vi "一个反馈计算误差.vi"(6 "第几组":i32, 7 "选择?":bool[](array[boolean]), 8 "设定值_2":dbl, 9 "设定值_1":dbl, 10 "反馈值_2":dbl, 11 "反馈值_1":dbl) -> (0 "字符串_误差_2":string, 1 "误差_2":dbl, 2 "字符串_误差_1":string, 3 "误差_1":dbl, 4 "合格_2?":bool, 5 "合格_1?":bool)   [LabVIEW 2010]
uses:
  全局量/全局_配置.vi
panel:
  # "0~31"
  # "0~15"
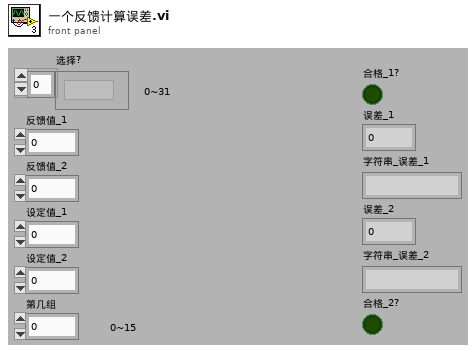
[diagram p1: front panel]
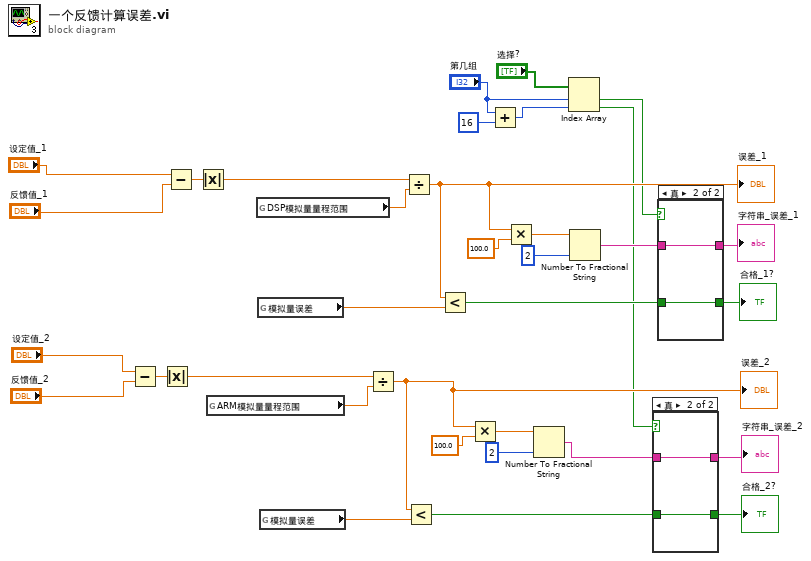
[diagram p0: block diagram]
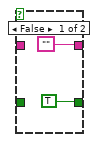
[diagram p2: hidden frame]
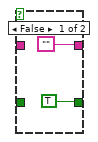
[diagram p3: hidden frame]
diagram:
  n1 = Subtract(x="设定值_2", y="反馈值_2") -> (x-y=w19:dbl)
  n2 = Absolute Value(x=w19) -> (abs(x)=w20:dbl)
  n3 = Subtract(x="设定值_1", y="反馈值_1") -> (x-y=w34:dbl)
  n4 = Absolute Value(x=w34) -> (abs(x)=w32:dbl)
  n5 = global read "全局_配置.vi" "ARM模拟量量程范围"() -> (w18:dbl)
  n6 = global read "全局_配置.vi" "DSP模拟量量程范围"() -> (w31:dbl)
  n7 = global read "全局_配置.vi" "模拟量误差"() -> (w30:dbl)
  n8 = global read "全局_配置.vi" "模拟量误差"() -> (w21:dbl)
  n9 = Divide(x=w20, y=w18) -> (x/y=w6:dbl)
  "误差_2" <- w6
  n10 = Divide(x=w32, y=w31) -> (x/y=w26:dbl)
  "误差_1" <- w26
  n11 = Less?(x=w6, y=w21) -> (x < y?=w2:bool)
  n12 = Less?(x=w26, y=w30) -> (x < y?=w8:bool)
  n13 = Multiply(x=w6, y=100.0) -> (x*y=w24:dbl)
  n14 = Add(x="第几组", y=16) -> (x+y=w12:i32)
  n15 = Multiply(x=w26, y=100.0) -> (x*y=w27:dbl)
  n16 = Number To Fractional String(number=w24, precision (6)=i16 2 ("精度(6)")) -> (F-format string=w5:string)  [unwired: 2 in]
  n17 = Index Array(array="选择?", index #1="第几组", index #2=w12) -> (element #1=w11:bool, element #2=w3:bool)
  n18 = Number To Fractional String(number=w27, precision (6)=i16 2 ("精度(6)")) -> (F-format string=w10:string)  [unwired: 2 in]
  n19 = case shown="真" w3 {
    tunnel: w5 -> [_ w38]
    tunnel: ["" w38] -> w4
    tunnel: w2 -> [_ w37]
    tunnel: [TRUE w37] -> w1
    frame False {
    }
    frame True {
    }
  }
  "字符串_误差_2" <- w4
  "合格_2?" <- w1
  n20 = case shown="真" w11 {
    tunnel: w10 -> [_ w42]
    tunnel: ["" w42] -> w9
    tunnel: w8 -> [_ w41]
    tunnel: [TRUE w41] -> w7
    frame False {
    }
    frame True {
    }
  }
  "合格_1?" <- w7
  "字符串_误差_1" <- w9
